vi "Read Pulse Width.vi"(8 "error in":errorcluster, 11 "DIG_IO in":refnum<class "DIG_IO.lvclass">) -> (0 "error out":errorcluster, 2 "Period":dbl, 3 "DIG_IO out":refnum<class "DIG_IO.lvclass">)   [LabVIEW 2019, in "DIG_IO.lvlib" / "DIG_IO.lvclass"]
uses:
  Library/DIG_IO.lvclass
  Library/DIG_IO.lvclass/DIG_IO.ctl
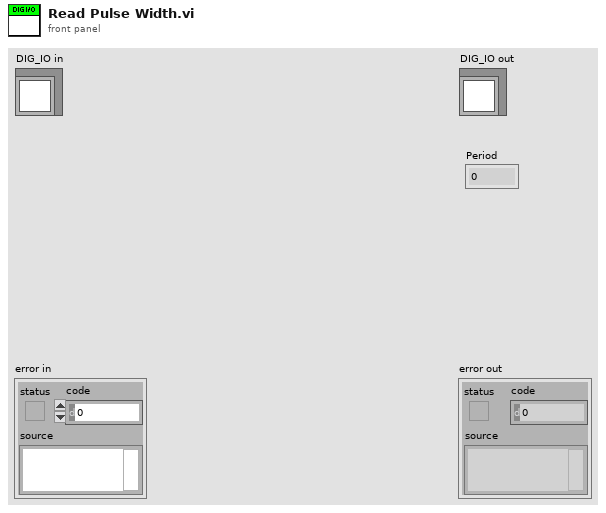
[diagram p1: front panel]
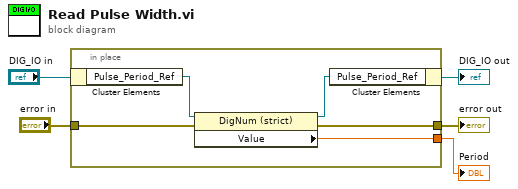
[diagram p0: block diagram]
diagram:
  n1 = in-place {
    in-place-border: "error in" -> [w8]
    in-place-border: [w7] -> w2
    in-place-border: [w6] -> w1
    n2 = in-place-cluster #1("DIG_IO in") -> ("Pulse_Period_Ref"=w10:refnum<vi>)
    n3 = property class="DigNum (strict)"(reference=w10, error in=w8) -> (reference out=w9:refnum<vi>, error out=w7:errorcluster, "Value"=w6:dbl)
    n4 = in-place-cluster #1("Pulse_Period_Ref"=w9) -> (→"DIG_IO out":refnum<class "DIG_IO.lvclass">)
  }
  "error out" <- w2
  "Period" <- w1
